vi "Find Missing Hardware Identifiers.vi"(8 "error in":errorcluster, 10 "validation information in":T1={"Missing Modules"=variant(cluster{"ID":string, "Path":string}[] []), "Module Connection Map"=variant, "Unused Modules"=variant(cluster{"ID":string, "Path":string}[] [])}, 11 "routing and faulting in":T2 format="%.0x") -> (0 "error out":errorcluster, 1 "identifier errors":errorcluster[](array[cluster]), 2 "validation information out":T1={"Missing Modules"=variant(cluster{"ID":string, "Path":string}[] []), "Module Connection Map"=variant, "Unused Modules"=variant(cluster{"ID":string, "Path":string}[] [])}, 3 "routing and faulting out":T2 format="%.0x")   [LabVIEW 2020, in "Routing and Faulting Scripting.lvlib"]
uses:
  Routing and Faulting Scripting.lvlib
  <vilib>/NI VeriStand/Custom Device API/Custom Device Item Ref.ctl
  Validation Information.ctl
  NationalInstruments.VeriStand.SystemStorage
  Constants/Scripting Constants.vi
  <vilib>/NI VeriStand/Custom Device API/Custom Device API.lvlib
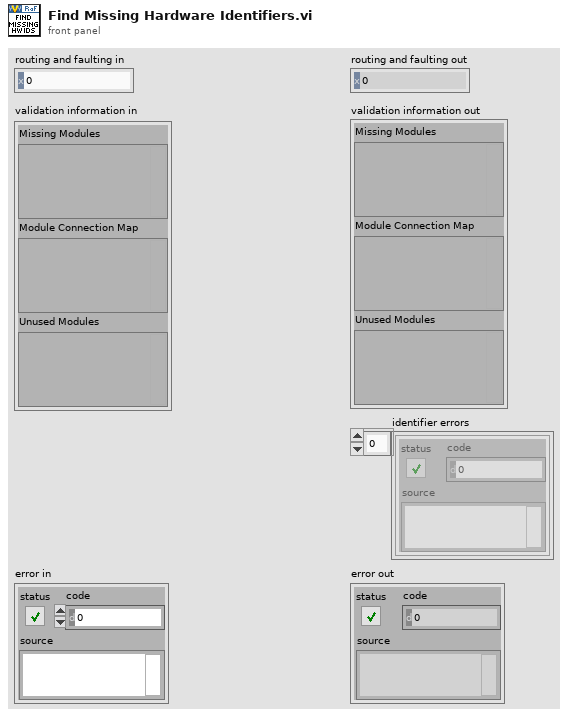
[diagram p1: front panel]
types:
  T1 = typedef "Routing and Faulting Scripting.lvlib/Validation Information.ctl" = cluster{"Missing Modules":variant, "Module Connection Map":variant, "Unused Modules":variant}
  T2 = typedef "Custom Device API.lvlib/Custom Device Item Ref.ctl" = u64
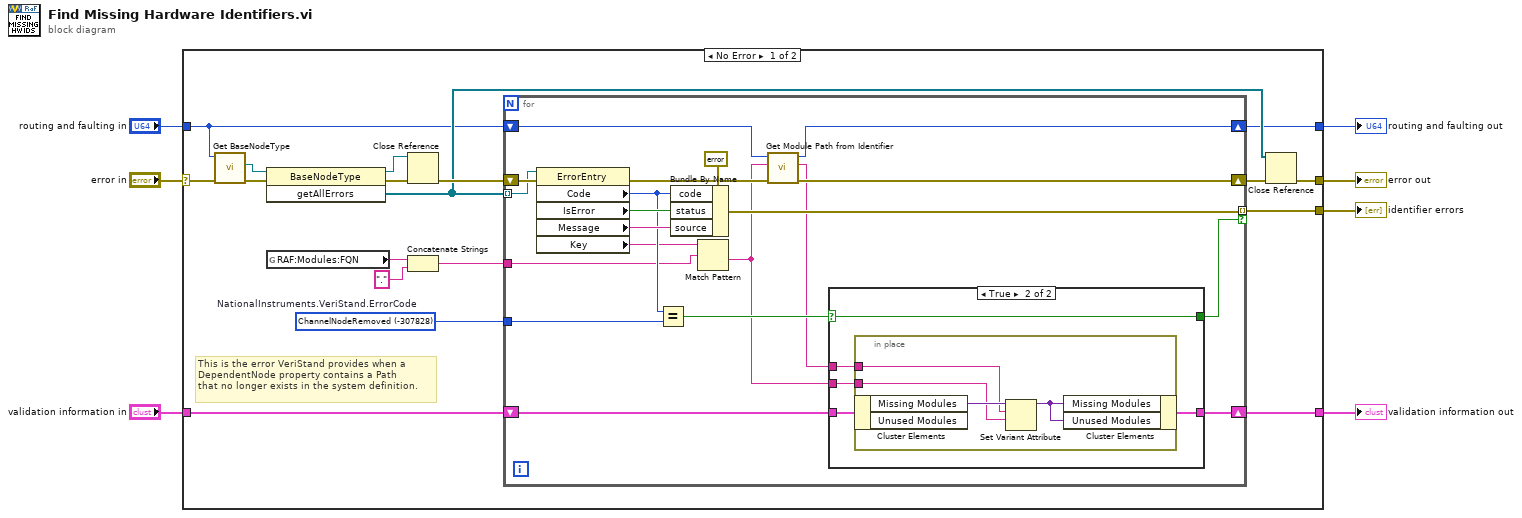
[diagram p0: block diagram]
diagram:
  n1 = case shown="No Error" "error in" {
    selector: "error in" -> [w17 w58]
    tunnel: "routing and faulting in" -> [w11 w59]
    tunnel: [w10 w59] -> w5
    tunnel: [w16 w58] -> w4
    tunnel: [w15 _] -> w3
    tunnel: "validation information in" -> [w9 w57]
    tunnel: [w8 w57] -> w1
    frame No Error {
      w19 = -307828 items=["Success"=0, "NoProjectOpen"=-307992, "SequenceCompileError"=-307988, "SessionAlreadyDeployed"=-307984, "SessionNotDeployed"=-307982, "SequenceNotFoundInSession"=-307981, "StimulusProfileSessionLocked"=-307980, "EmptyNodeName"=-307930, "NodeAlreadyExistsByName"=-307926, "NumberOfCoefficientsOutOfRange"=-307884, "DownloadFileError"=-307872, "IncorrectLogFileName"=-307871, "LogTriggerConditionSyntaxError"=-307868, "DuplicateLogSessionName"=-307867, "LogSessionNotFound"=-307865, "ChannelLengthMismatch"=-307830, "NodeNotFoundDuringCompile"=-307829, "ChannelNodeRemoved"=-307828, "NotAChannel"=-307825, "NotAWaveform"=-307824, "STIFileError"=-307784, "DependenciesCycle"=-307783, "ChannelNotFoundInLogFile"=-307782, "ChannelGroupNotFoundInLogFile"=-307781, "GatewayNotOnLocalhost"=-307780, "NotEnoughDynamicDataSharingSpace"=-307738, "TargetMissingDataSharingDevice"=-307737, "ChannelMappingsSizeMismatch"=-307728, "DuplicateChannelAliasMappings"=-307711, "NotAnInlineCustomDevice"=-307710, "IncompatibleModel"=-307703, "ModelDimensionMismatch"=-307702, "SLSCChassisLoadFailed"=-307691, "TargetDisabled"=-307689, "MismatchedLengths"=-307687, "TargetInvalid"=-307686, "ParameterNotFound"=-307685, "ServerPortAlreadyInUse"=-307684, "TargetDisconnected"=-307682, "ServiceConfigurationFile"=-307681, "ModelParameterFileParseError"=-307680, "NoActionRequired"=-307677, "InputParameterInvalid"=-307676, "HostRunningDifferentSystemDefinition"=-307671, "ChannelNotScalable"=-307668, "ChannelCannotBeFaulted"=-307666, "ChannelNotWritable"=-307665, "ChannelNotReadable"=-307664, "Timeout"=-307663, "NodeNotFound"=-307662, "SystemDefinitionDeploymentFailure"=-307661, "SystemDefinitionDeploymentTimeout"=-307660, "EmptyPassword"=-307659, "SystemDefinitionAlreadyActive"=-307658, "InvalidConfigurationPassword"=-307657, "NoSystemDefinitionLoaded"=-307656, "ComponentNotAvailable"=-307655, "NotDeployed"=-307654, "InvalidFile"=-307653, "FailedServerConnection"=-307652, "FunctionNotSupported"=-307651, "UnexpectedError"=-307650, "UnmappedAlias"=-307617, "InvalidStreamConditionForDataType"=-307554, "WaveformDataTypeMismatch"=-307553, "InvalidDaqPluginFile"=-307526, "FileVersionUnsupported"=-307525]  # NationalInstruments.VeriStand.ErrorCode
      # "This is the error VeriStand provides when a\nDependentNode property contains a Path\nthat no longer exists in the system definition."
      n2 = call "Get BaseNodeType.vi"("error in"=w17, "item in"=w11) -> ("error out"=w25:errorcluster, "BaseNodeType"=w24:refnum<k24>)  [unwired: 7 in, 1 out]
      n3 = invoke class="BaseNodeType" method="getAllErrors"(reference=w24, error in=w25) -> (reference out=w22:refnum<k24>, error out=w23:errorcluster, "getAllErrors"=w18:refnum<k24>[])  [unwired: 1 in]
      n4 = global read "Scripting Constants.vi" "RAF:Modules:FQN"() -> (w14:string)
      n5 = Close Reference(reference=w22, error in (no error)=w23) -> (error out=w21:errorcluster)
      n6 = Concatenate Strings(w14, "." ("string")) -> (w12:string)
      n7 = for {
        shift-right: [w32] -> w20
        shift-left: w21 -> [w45]
        tunnel: w18 -> [w44] mode=indexing
        tunnel: [w40] -> w15 mode=indexing if=w26
        tunnel: w19 -> [w39]
        tunnel: w12 -> [w36]
        shift-right: [w33] -> w10
        shift-left: w11 -> [w34]
        shift-right: [w29] -> w8
        shift-left: w9 -> [w31]
        n8 = property class="ErrorEntry"(reference=w44, error in=w45) -> (error out=w35:errorcluster, "Code"=w38:i32, "IsError"=w42:bool, "Message"=w41:string, "Key"=w37:string)  [unwired: 1 out]
        n9 = Equal?(x=w38, y=w39) -> (x = y?=w30:bool)
        n10 = Bundle By Name(cluster=errorcluster {"status"=FALSE, "code"=0, "source"=""} ("error out"), "code"=w38, "status"=w42, "source"=w41) -> (w40:errorcluster)
        n11 = Match Pattern(string=w37, regular expression=w36) -> (after substring=w28:string)  [unwired: 1 in, 3 out]
        n12 = call "Get Module Path from Identifier.vi"("error in"=w35, "module identifier"=w28, "routing and faulting in"=w34) -> ("error out"=w32:errorcluster, "module path"=w27:string, "routing and faulting out"=w33:T2)  [unwired: 6 in]
        n13 = case shown="True" w30 {
          selector: w30 -> [w46 w48]
          tunnel: w31 -> [w47 w52]
          tunnel: [w47 w51] -> w29
          tunnel: w28 -> [_ w50]
          tunnel: w27 -> [_ w49]
          tunnel: [w46 w48] -> w26
          frame False {
          }
          frame True {
            n14 = in-place {
              in-place-border: w50 -> [w54]
              in-place-border: w49 -> [w53]
              n15 = in-place-cluster #1(w52) -> ("Missing Modules"=w56:variant)  [unwired: 1 out]
              n16 = Set Variant Attribute(Variant=w56, name=w53, value=w54) -> (Variant out=w55:variant)  [unwired: 1 in, 2 out]
              n17 = in-place-cluster #1("Missing Modules"=w55, "Unused Modules"=w55) -> (w51:T1)
            }
          }
        }
      }
      n18 = Close Reference(reference=w18, error in (no error)=w20) -> (error out=w16:errorcluster)
    }
    frame Error {
    }
  }
  "routing and faulting out" <- w5
  "error out" <- w4
  "identifier errors" <- w3
  "validation information out" <- w1
